vi "CAENInit.vi"(0 "IP Address":string, 4 "error in (no error)":errorcluster) -> (8 "Power Supply Response":string, 9 "Output Cluster":T2 {"MaxLambdaCurrent [A]" format="%.2f"; "LambdaRates [A/min]" format="%.5e"; "MaxNormalCurrent [A]" format="%.2f"; "StabilitySetting [%]" format="%.2f"; "FieldCurrentRatio [T/A]" format="%.2f"; "SwitchWaitTime [s]" format="%.2f"; "SwitchHtrCurrent [mA]" format="%.2f"; "TrainRates [A/min]" format="%.5e"; "NormalRates [A/min]" format="%.5e"; "Breakpts [A]" format="%.5e"}, 11 "error out":errorcluster, 12 "Network Session Out":refnum<k5>, 13 "Mode Out":T1(ring), 14 "Current Set Point":dbl, 15 "Actual Ouput Current":dbl, 16 "Current Slew Rate (A/s)":dbl, 17 "Field Set Point":dbl, 18 "Actual Field":dbl, 19 "Field Ramp Rate (T/min)":dbl)   [LabVIEW 2025]
doc: "Author: Scott Hannahs <sth@magnet.fsu.edu>\n\nThis software is licensed for use under the “MIT License\"\nCopyright (c) 2025 Scott Hannahs, sth@sth@magnet.sthnet.net\n\nPermission is hereby granted, free of charge, to any person obtaining a copy of this software and associated documentation files (the \"Software\"), to deal in the Software without restriction, including without limitation the rights to use, copy, modify, merge, publish, distribute, sublicense, and/or sell copies of the Software, and to permit persons to whom the Software is furnished to do so, subject to the following conditions: The above copyright notice and this permission notice shall be included in all copies or substantial portions of the Software.\n\nTHE SOFTWARE IS PROVIDED \"AS IS\", WITHOUT WARRANTY OF ANY KIND, EXPRESS OR IMPLIED, INCLUDING BUT NOT LIMITED TO THE WARRANTIES OF MERCHANTABILITY, FITNESS FOR A PARTICULAR PURPOSE AND NONINFRINGEMENT. IN NO EVENT SHALL THE AUTHORS OR COPYRIGHT HOLDERS BE LIABLE FOR ANY CLAIM, DAMAGES OR OTHER LIABILITY, WHETHER IN AN ACTION OF CONTRACT, TORT OR OTHERWISE, ARISING FROM, OUT OF OR IN CONNECTION WITH THE SOFTWARE OR THE USE OR OTHER DEALINGS IN THE SOFTWARE."
uses:
  VISA stuff/Misc Extras/Manufacturer Drivers/Caens PS LabVIEW Driver/Driver/CAENels FAST-PS.lvlib
panel:
  in  "Input Cluster":T2 {"MaxLambdaCurrent [A]" format="%.2f"; "LambdaRates [A/min]" format="%.5e"; "MaxNormalCurrent [A]" format="%.2f"; "StabilitySetting [%]" format="%.2f"; "FieldCurrentRatio [T/A]" format="%.2f"; "SwitchWaitTime [s]" format="%.2f"; "SwitchHtrCurrent [mA]" format="%.2f"; "TrainRates [A/min]" format="%.5e"; "NormalRates [A/min]" format="%.5e"; "Breakpts [A]" format="%.5e"}
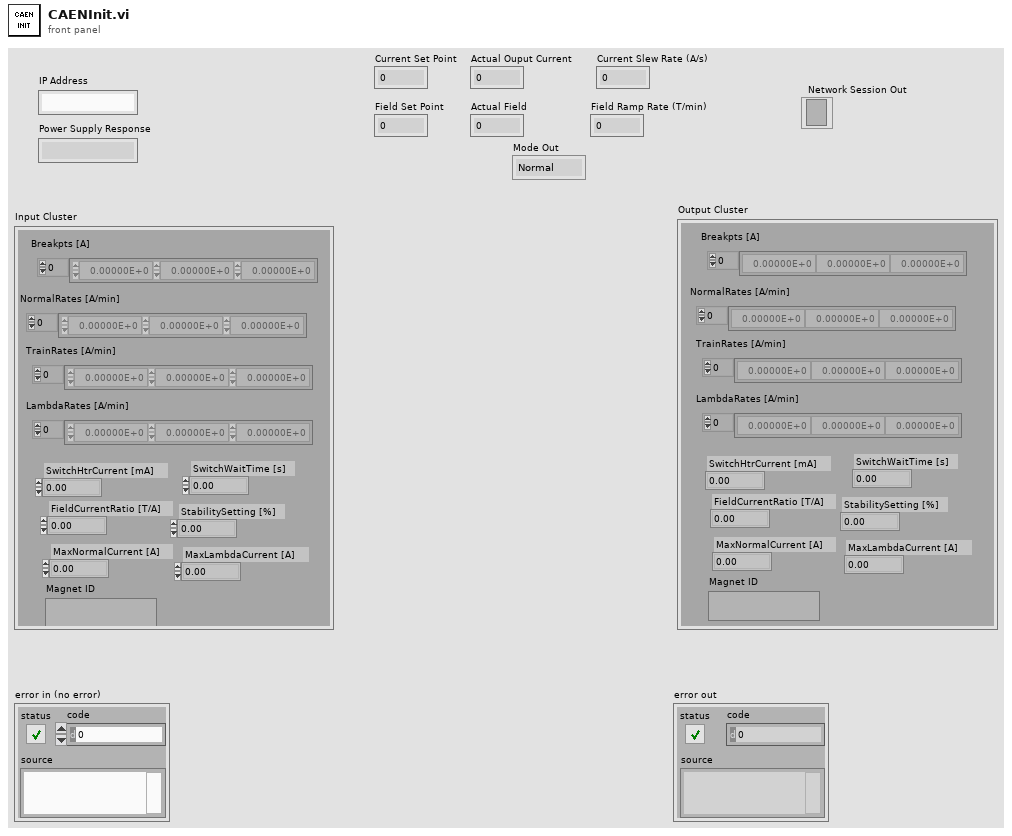
[diagram p1: front panel]
types:
  T1 = enum16{"Normal", "Train", "Lambda", "Train & Lambda"}
  T2 = cluster{"Breakpts [A]":dbl[], "NormalRates [A/min]":dbl[], "TrainRates [A/min]":dbl[], "SwitchHtrCurrent [mA]":dbl, "SwitchWaitTime [s]":dbl, "FieldCurrentRatio [T/A]":dbl, "StabilitySetting [%]":dbl, "MaxNormalCurrent [A]":dbl, "Magnet ID":string, "LambdaRates [A/min]":dbl[], "MaxLambdaCurrent [A]":dbl}
  T3 = enum16{"Paused", "Ramping to Programmed Field", "QUENCH"}
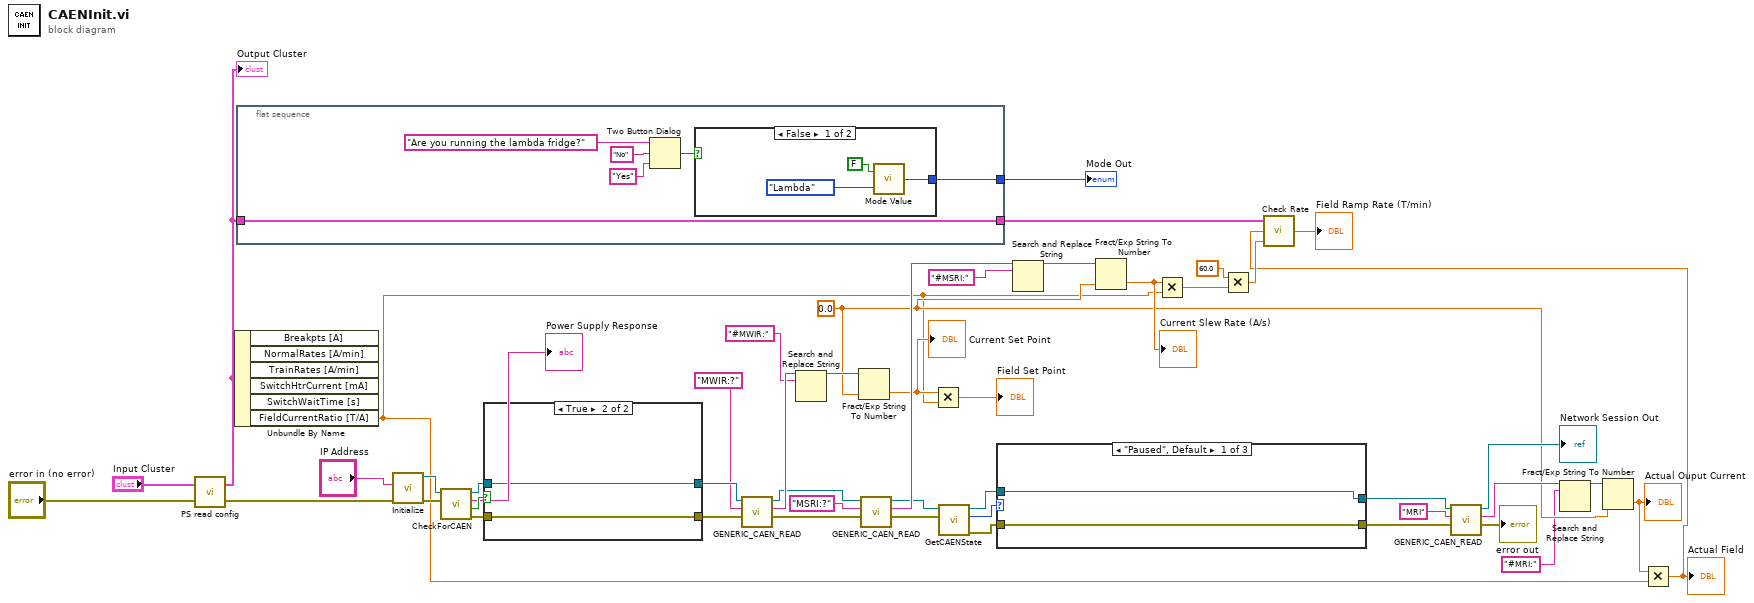
[diagram p0: block diagram]
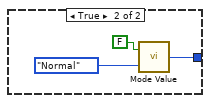
[diagram p2: hidden frame]
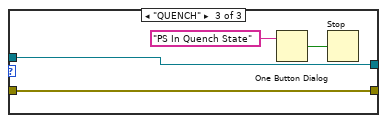
[diagram p4: hidden frame]
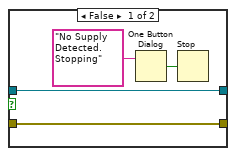
[diagram p5: hidden frame]
diagram:
  w14 = 0.0
  n1 = call "PS read config.vi"("error in (no error)"="error in (no error)", "Input Cluster"="Input Cluster") -> ("error out"=w6:errorcluster, "output cluster"=w9:T2)
  "Output Cluster" <- w9
  n2 = Unbundle By Name(w9) -> ("FieldCurrentRatio [T/A]"=w12:dbl)  [unwired: 5 out]
  n3 = flat-sequence {
    tunnel: [w51] -> w10
    tunnel: w9 -> [w50]
    tunnel: [w50] -> w8
    frame #0 {
      n4 = Two Button Dialog(message="Are you running the lambda fridge?", 1:"Yes", 2:"No") -> (T button?=w52:bool)
      n5 = case shown="False" w52 {
        tunnel: [w56 w60] -> w51
        frame False {
          n6 = call "Mode Value.vi"("Mode In"=T1."Lambda" ("Mode Out"), "Read/Write this vi"=FALSE) -> ("Mode Out"=w56:T1)
        }
        frame True {
          n7 = call "Mode Value.vi"("Mode In"=T1."Normal" ("Mode Out"), "Read/Write this vi"=FALSE) -> ("Mode Out"=w60:T1)
        }
      }
    }
  }
  n8 = call "Initialize.vi"("error in (no error)"=w6, "IP address"="IP Address") -> ("error out"=w47:errorcluster, "connection ID"=w48:refnum<k5>)  [unwired: 4 in]
  n9 = call "CheckForCAEN.vi"("error in"=w47, "Network Session"=w48) -> ("error out"=w45:errorcluster, "Boolean"=w46:bool, "String"=→"Power Supply Response":string, "TCP Network Connection Refnum"=w44:refnum<k5>)  [unwired: 6 in]
  n10 = case shown="True" w46 {
    tunnel: w45 -> [w65 w67]
    tunnel: [w65 w67] -> w42
    tunnel: w44 -> [w64 w66]
    tunnel: [w64 w66] -> w43
    frame False {
      n11 = One Button Dialog(message="No Supply Detected. Stopping") -> (true=w62:bool)  [unwired: 1 in]
      n12 = Stop(stop? (T)=w62) -> ()
    }
    frame True {
    }
  }
  n13 = call "GENERIC_CAEN_READ.vi"("error in (no error)"=w42, "String"="MWIR:?", "Network Session"=w43) -> ("error out"=w36:errorcluster, "String 2"=w41:string, "Network Session Out"=w37:refnum<k5>)  [unwired: 6 in]
  n14 = Search and Replace String(input string=w41, search string="#MWIR:") -> (result string=w39:string)  [unwired: 6 in, 3 out]
  n15 = Fract/Exp String To Number(string=w39, default (0 dbl)=w14) -> (number=w27:dbl)  [unwired: 2 in, 1 out]
  "Current Set Point" <- w27
  n16 = call "GENERIC_CAEN_READ.vi"("error in (no error)"=w36, "String"="MSRI:?", "Network Session"=w37) -> ("error out"=w31:errorcluster, "String 2"=w35:string, "Network Session Out"=w32:refnum<k5>)  [unwired: 6 in]
  n17 = Multiply(x=w27, y=w12) -> (x*y=→"Field Set Point":dbl)
  n18 = call "GetCAENState.vi"("error in (no error)"=w31, "TCP Session"=w32) -> ("error out"=w2:errorcluster, "Enum"=w29:T3, "TCP Session Out"=w30:refnum<k5>)  [unwired: 6 in, 1 out]
  n19 = case shown="\"Paused\", Default" w29 {
    tunnel: w30 -> [w69 w71 w75]
    tunnel: [w69 w71 w75] -> w20
    tunnel: w2 -> [w68 w70 w72]
    tunnel: [w68 w70 w72] -> w19
    frame "Paused", Default {
    }
    frame "Ramping to Programmed Field" {
    }
    frame "QUENCH" {
      n20 = One Button Dialog(message="PS In Quench State") -> (true=w74:bool)  [unwired: 1 in]
      n21 = Stop(stop? (T)=w74) -> ()
    }
  }
  n22 = Search and Replace String(input string=w35, search string="#MSRI:") -> (result string=w33:string)  [unwired: 6 in, 3 out]
  n23 = Fract/Exp String To Number(string=w33, default (0 dbl)=w14) -> (number=w25:dbl)  [unwired: 2 in, 1 out]
  "Current Slew Rate (A/s)" <- w25
  n24 = Multiply(x=w25, y=w12) -> (x*y=w24:dbl)
  n25 = Multiply(x=60.0, y=w24) -> (x*y=w22:dbl)
  n26 = call "GENERIC_CAEN_READ.vi"("error in (no error)"=w19, "String"="MRI", "Network Session"=w20) -> ("error out"=→"error out":errorcluster, "String 2"=w16:string, "Network Session Out"=→"Network Session Out":refnum<k5>)  [unwired: 6 in]
  n27 = Search and Replace String(input string=w16, search string="#MRI:") -> (result string=w15:string)  [unwired: 6 in, 3 out]
  n28 = Fract/Exp String To Number(string=w15, default (0 dbl)=w14) -> (number=w11:dbl)  [unwired: 2 in, 1 out]
  "Actual Ouput Current" <- w11
  n29 = Multiply(x=w11, y=w12) -> (x*y=w4:dbl)
  "Actual Field" <- w4
  n30 = call "Check Rate.vi"("Rate"=w22, "Field"=w4, "input cluster"=w8) -> ("Checked Rate"=→"Field Ramp Rate (T/min)":dbl)
  "Mode Out" <- w10
